vi "Set Error Reporting.vi"(8 "error in (no error)":errorcluster, 10 "Error Reporting":T1, 11 "DeviceComms in":refnum<class "DeviceComms.lvclass">) -> (0 "error out":errorcluster, 3 "DeviceComms out":refnum<class "DeviceComms.lvclass">)   [LabVIEW 2020, in "CTI.lvlib" / "DeviceComms.lvclass"]
uses:
  DeviceComms.lvclass
  Error Reporting.ctl
  CTI.lvlib
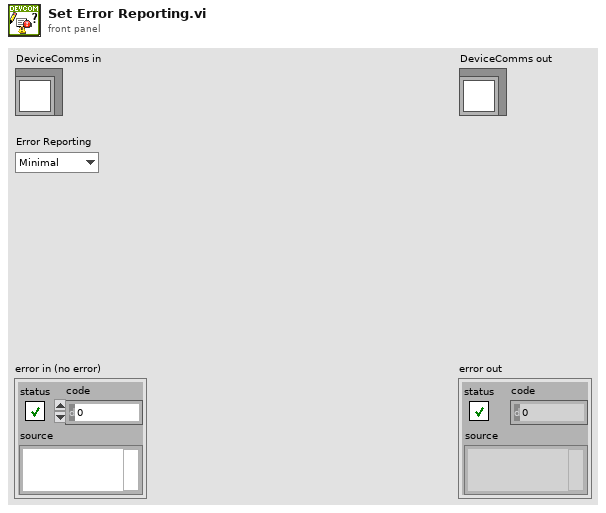
[diagram p1: front panel]
types:
  T1 = typedef "CTI.lvlib/Error Reporting.ctl" = enum16{"Minimal", "Moderate", "Full"}
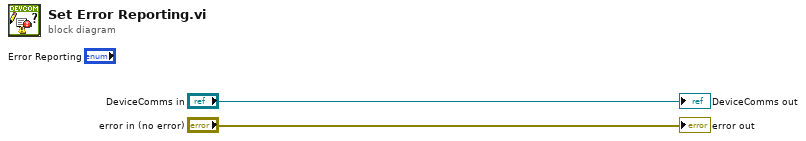
[diagram p0: block diagram]
diagram:
  "error out" <- "error in (no error)"
  "DeviceComms out" <- "DeviceComms in"
